vi "Encode.vi"   [LabVIEW 2020, in "feature_detection.lvlib" / "QR Code Encoder.lvclass"]
doc: "Encode the supplied Data into QR Code Image Data."
uses:
  QR Code Encoder.lvclass
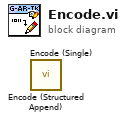
[diagram p0: block diagram]
diagram:
  n1 = call "Encode (Structured Append).vi"() -> ()  [unwired: 9 in, 3 out]
  n2 = call "Encode (Single).vi"() -> ()  [unwired: 9 in, 3 out]
